vi "GasteilerInListeFinden.vi"(10 "Gasteiler definition":T1 {"Gasteiler Letzte Wartung" format="%<%x %.3X>T"}, 11 "GasteilerListe":T1[](array[typedef]) {"Gasteiler Letzte Wartung" format="%<%x %.3X>T"}) -> (1 "gefunden":bool, 2 "Index":i32, 3 "GasteilerListe out":T1[](array[typedef]) {"Gasteiler Letzte Wartung" format="%<%x %.3X>T"})   [LabVIEW 2020, in "System Einstellungen V2.lvlib"]
uses:
  Gasteiler.ctl
  System Einstellungen V2.lvlib
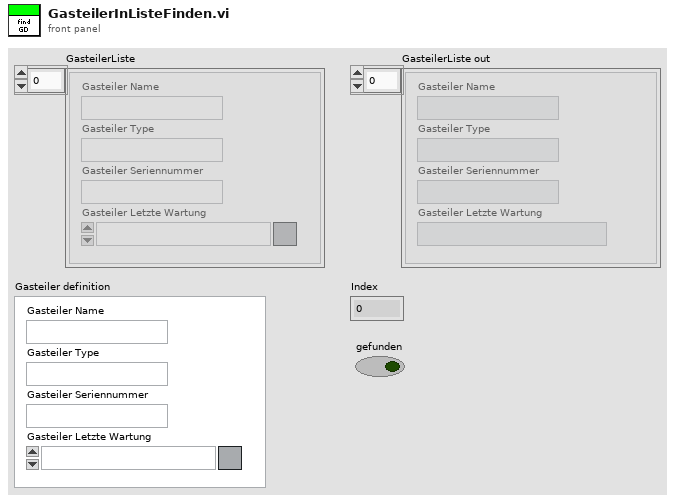
[diagram p1: front panel]
types:
  T1 = typedef "System Einstellungen V2.lvlib/Gasteiler.ctl" = cluster{"Gasteiler Name":string, "Gasteiler Type":string, "Gasteiler Seriennummer":string, "Gasteiler Letzte Wartung":timestamp}
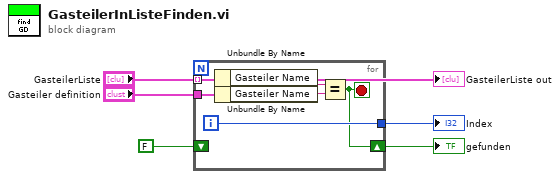
[diagram p0: block diagram]
diagram:
  n1 = for {
    tunnel: "Gasteiler definition" -> [w10]
    tunnel: "GasteilerListe" -> [w11] mode=indexing
    tunnel: [w7] -> w4
    shift-right: [w6] -> w1
    shift-left: FALSE -> [_]
    i -> [w7]
    stop <- w6 stop-if-true
    n2 = Unbundle By Name(w11) -> ("Gasteiler Name"=w9:string)
    n3 = Unbundle By Name(w10) -> ("Gasteiler Name"=w8:string)
    n4 = Equal?(x=w9, y=w8) -> (x = y?=w6:bool)
  }
  "Index" <- w4
  "gefunden" <- w1
  "GasteilerListe out" <- "GasteilerListe"
